vi "midi_value.from_enum.vi"(10 "MIDI Status Byte":T1) -> (2 "midi status value":u8)   [LabVIEW 2020, in "MIDIllan.lvlib"]
uses:
  MIDIllan.lvlib
  midi status byte.ctl
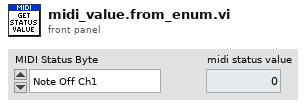
[diagram p1: front panel]
types:
  T1 = typedef "MIDIllan.lvlib/midi status byte.ctl" = enum8{"Note Off Ch1", "Note Off Ch2", "Note Off Ch3", "Note Off Ch4", "Note Off Ch5", "Note Off Ch6", "Note Off Ch7", "Note Off Ch8", "Note Off Ch9", "Note Off Ch10", "Note Off Ch11", "Note Off Ch12", "Note Off Ch13", "Note Off Ch14", "Note Off Ch15", "Note Off Ch16", "Note On Ch1", "Note On Ch2", "Note On Ch3", "Note On Ch4", "Note On Ch5", "Note On Ch6", "Note On Ch7", "Note On Ch8", "Note On Ch9", "Note On Ch10", "Note On Ch11", "Note On Ch12", "Note On Ch13", "Note On Ch14", "Note On Ch15", "Note On Ch16", "Poly Aftertouch Ch1", "Poly Aftertouch Ch2", "Poly Aftertouch Ch3", "Poly Aftertouch Ch4", "Poly Aftertouch Ch5", "Poly Aftertouch Ch6", "Poly Aftertouch Ch7", "Poly Aftertouch Ch8", "Poly Aftertouch Ch9", "Poly Aftertouch Ch10", "Poly Aftertouch Ch11", "Poly Aftertouch Ch12", "Poly Aftertouch Ch13", "Poly Aftertouch Ch14", "Poly Aftertouch Ch15", "Poly Aftertouch Ch16", "Control Change Ch1", "Control Change Ch2", "Control Change Ch3", "Control Change Ch4", "Control Change Ch5", "Control Change Ch6", "Control Change Ch7", "Control Change Ch8", "Control Change Ch9", "Control Change Ch10", "Control Change Ch11", "Control Change Ch12", "Control Change Ch13", "Control Change Ch14", "Control Change Ch15", "Control Change Ch16", "Program Change Ch1", "Program Change Ch2", "Program Change Ch3", "Program Change Ch4", "Program Change Ch5", "Program Change Ch6", "Program Change Ch7", "Program Change Ch8", "Program Change Ch9", "Program Change Ch10", "Program Change Ch11", "Program Change Ch12", "Program Change Ch13", "Program Change Ch14", "Program Change Ch15", "Program Change Ch16", "Channel Aftertouch Ch1", "Channel Aftertouch Ch2", "Channel Aftertouch Ch3", "Channel Aftertouch Ch4", "Channel Aftertouch Ch5", "Channel Aftertouch Ch6", "Channel Aftertouch Ch7", "Channel Aftertouch Ch8", "Channel Aftertouch Ch9", "Channel Aftertouch Ch10", "Channel Aftertouch Ch11", "Channel Aftertouch Ch12", "Channel Aftertouch Ch13", "Channel Aftertouch Ch14", "Channel Aftertouch Ch15", "Channel Aftertouch Ch16", "Pitch Bend Ch1", "Pitch Bend Ch2", "Pitch Bend Ch3", "Pitch Bend Ch4", "Pitch Bend Ch5", "Pitch Bend Ch6", "Pitch Bend Ch7", "Pitch Bend Ch8", "Pitch Bend Ch9", "Pitch Bend Ch10", "Pitch Bend Ch11", "Pitch Bend Ch12", "Pitch Bend Ch13", "Pitch Bend Ch14", "Pitch Bend Ch15", "Pitch Bend Ch16", "System Exclusive Start", "MIDI Time Code Quarter Frame", "Song Position Pointer", "Song Select", "System Common Undefined F4", "System Common Undefined F5", "Tune Request", "System Exclusive End", "Timing Clock", "System Real-time Undefined F9", "Start", "Continue", "Stop", "System Real-time Undefined FD", "Active Sensing", "System Reset"}
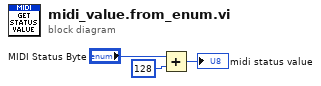
[diagram p0: block diagram]
diagram:
  n1 = Add(x="MIDI Status Byte", y=128) -> (x+y=→"midi status value":i32)
